vi "Wait Return.vi"(8 "entrée d'erreur (pas d'erreur)":errorcluster, 10 "Report ?":bool, 11 "Send_Frame en entrée":refnum<class "Nodon_Send_Command_UART.lvclass">) -> (0 "sortie d'erreur":errorcluster, 1 "Send again":bool, 2 "Data":string, 3 "Send_Frame en sortie":refnum<class "Nodon_Send_Command_UART.lvclass">, 4 "Command ID":string, 5 "Command Type":string)   [LabVIEW 2020, in "Library Test.lvlib" / "Nodon_Send_Command_UART.lvclass"]
uses:
  Nodon_Send_Command_UART.lvclass
  C:/Users/ngarcin/OneDrive - Altyor/Standard TB/Class/Test/Test (Default)/Test (Default).lvclass
  Commun VI/TypeDef/Commande UART/Parametre UART.ctl
  UART/UART (Default)/Class UART (Default).lvclass
  JSON API/JSON Value/Set from JSON string.vi
  JSON API/Variant JSON/Variant to JSON.vi
  JSON API/JSON Value/Get Item by name array.vi
  Instrument/Instrument (Default)/Class Instrument (Default).lvclass
  JSON API/JSON Value/JSON Value.lvclass
  Nodon_Send_Command_UART.lvclass/Nodon_Send_Command_UART.ctl
  JSON API/Variant JSON/Variant JSON.lvlib
  JSON API/Get Polymorphic/JSON GetSet.lvlib
  Commun VI/Library Commun.lvlib
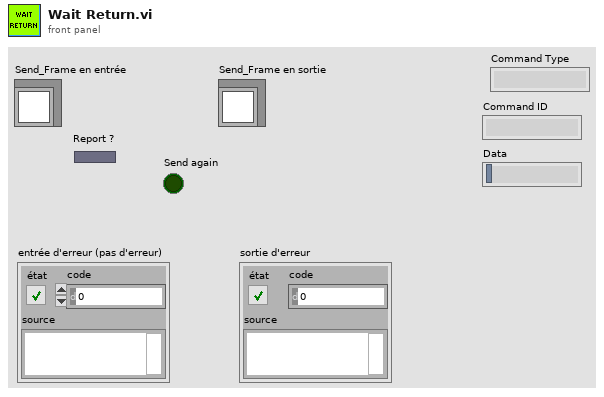
[diagram p1: front panel]
types:
  T1 = typedef "Parametre UART.ctl" = cluster{"Address Device":refnum<visa-resource-name>, "Baud Rate":u32, "Data Bit":u16, "stop bits (10: 1 bit)":u16, "parity (0:none)":enum16{"None", "Odd", "Even", "Mark", "Space"}, "flow control (0:none)":u16, "termination char ":u8, "Enable Termination":bool, "Nb Octet to Read":u16, "Class UART":refnum<class "Class UART (Default).lvclass">}
  T2 = cluster{"Frame Read":string, "Frame received":bool, "Frame NOk":bool}
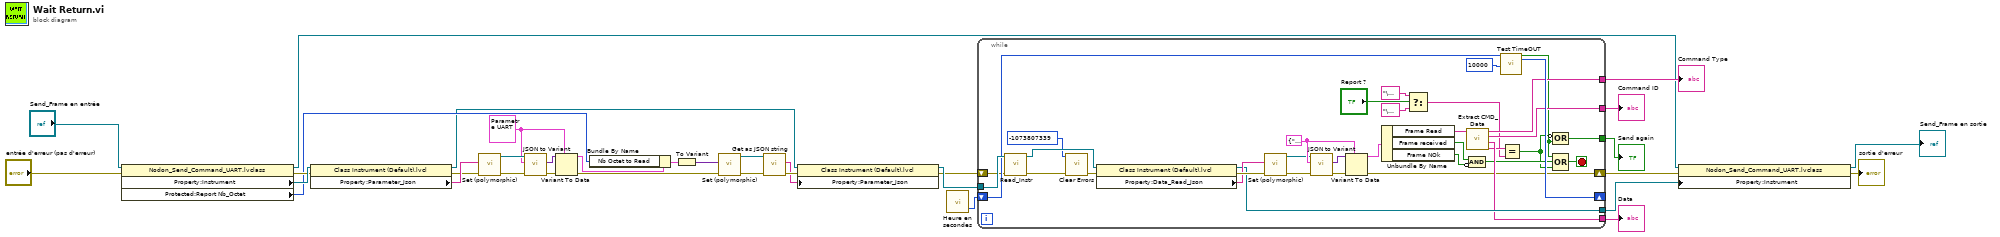
[diagram p0: block diagram]
diagram:
  w14 = T1 {"Address Device"="", "Baud Rate"=0, "Data Bit"=0, "stop bits (10: 1 bit)"=0, "parity (0:none)"=enum."None", "flow control (0:none)"=0, "termination char "=0, "Enable Termination"=FALSE, "Nb Octet to Read"=0, "Class UART"=refnum} ("Parameter")
  n1 = property class="Nodon_Send_Command_UART.lvclass"(reference="Send_Frame en entrée", error in="entrée d'erreur (pas d'erreur)") -> (reference out=w23:refnum<class "Nodon_Send_Command_UART.lvclass">, error out=w15:errorcluster, "Property:Instrument"=w16:refnum<class "Class Instrument (Default).lvclass">, "Protected:Report Nb_Octet"=w12:u16)
  n2 = property class="Class Instrument (Default).lvcl"(reference=w16, error in=w15) -> (reference out=w6:refnum<class "Class Instrument (Default).lvclass">, error out=w17:errorcluster, "Property:Parameter_Json"=w18:string)
  n3 = call-poly "Set (polymorphic).vi"("error in (no error)"=w17, "JSON stream"=w18) -> ("error out"=w20:errorcluster, "JSON Value out"=w22:refnum<class "JSON Value.lvclass">)  [unwired: 7 in, 1 out]
  n4 = call "JSON to Variant.vi"("error in (no error)"=w20, "Variant (Data Type)"=w14, "JSON Value"=w22) -> ("error out"=w21:errorcluster, "Variant out"=w19:variant)  [unwired: 7 in]
  n5 = Variant To Data(error in=w21, type=w14, Variant=w19) -> (data=w13:T1, error out=w8:errorcluster)
  n6 = Bundle By Name(cluster=w13, "Nb Octet to Read"=w12) -> (w7:T1)
  n7 = To Variant(anything=w7) -> (Variant=w11:variant)
  n8 = call-poly "Set (polymorphic).vi"("error in (no error)"=w8, "Variant"=w11) -> ("error out"=w9:errorcluster, "JSON Value out"=w10:refnum<class "JSON Value.lvclass">)  [unwired: 8 in]
  n9 = call "Get as JSON string.vi"("error in (no error)"=w9, "JSON Value in"=w10) -> ("error out"=w4:errorcluster, "<JSON>"=w2:string)  [unwired: 8 in]
  n10 = property class="Class Instrument (Default).lvcl"(reference=w6, error in=w4, "Property:Parameter_Json"=w2) -> (reference out=w5:refnum<class "Class Instrument (Default).lvclass">, error out=w3:errorcluster)
  n11 = call "Heure en secondes.vi"() -> ("Heure en milisecondes"=w1:u32)  [unwired: 2 in, 1 out]
  n12 = while {
    tunnel: w5 -> [w59]
    shift-right: [w50] -> w27
    shift-left: w3 -> [w37]
    tunnel: [w57] -> w24
    shift-right: [w55] -> _
    shift-left: w1 -> [w56]
    tunnel: [w51] -> w33
    tunnel: [w52] -> w32
    tunnel: [w49] -> w31
    tunnel: [w48] -> w30
    stop <- w45 stop-if-true
    w67 = T2 {"Frame Read"="", "Frame received"=FALSE, "Frame NOk"=FALSE}
    n13 = call-dynamic "Read_Instr.vi"("error in (no error)"=w37, "Class Instrument (Default) en entrée"=w59) -> ("error out"=w36:errorcluster, "Class Instrument (Default) en sortie"=w60:refnum<class "Class Instrument (Default).lvclass">)  [unwired: 8 in]
    n14 = call <vilib>:"Clear Errors.vi"("error in (no error)"=w36, "specific error code to clear (0: all)"=-1073807339) -> ("error out"=w34:errorcluster)  [unwired: 4 in, 1 out]
    n15 = property class="Class Instrument (Default).lvcl"(reference=w60, error in=w34) -> (reference out=w57:refnum<class "Class Instrument (Default).lvclass">, error out=w65:errorcluster, "Property:Data_Read_Json"=w64:string)
    n16 = call-poly "Set (polymorphic).vi"("error in (no error)"=w65, "JSON stream"=w64) -> ("error out"=w61:errorcluster, "JSON Value out"=w63:refnum<class "JSON Value.lvclass">)  [unwired: 7 in, 1 out]
    n17 = call "JSON to Variant.vi"("error in (no error)"=w61, "Variant (Data Type)"=w67, "JSON Value"=w63) -> ("error out"=w62:errorcluster, "Variant out"=w66:variant)  [unwired: 7 in]
    n18 = Variant To Data(error in=w62, type=w67, Variant=w66) -> (data=w68:T2, error out=w50:errorcluster)
    n19 = Unbundle By Name(w68) -> ("Frame Read"=w38:string, "Frame received"=w58:bool, "Frame NOk"=w54:bool)
    n20 = Select(t="\u0000" ("cas vrai"), s="Report ?", f="\u0001" ("x")) -> (s? t:f=w41:string)
    n21 = call "Extract CMD_Data.vi"("Frame"=w38) -> ("Frame Type"=w44:string, "DATA"=w51:string, "Command ID"=w49:string, "Command Type"=w48:string)  [unwired: 7 in]
    n22 = Compound Arithmetic op=AND ("Opérateur arithmétique")(w58, invert w54) -> (w47:bool)
    n23 = call "Test TimeOUT.vi"("OLD Time"=w56, "TimeOut ms"=u32 10000) -> ("Timeout ?"=w46:bool, "NEW Time"=w55:u32)  [unwired: 13 in, 3 out]
    n24 = Equal?(x=w44, y=w41) -> (x = y?=w39:bool)
    n25 = Compound Arithmetic op=OR ("Opérateur arithmétique")(invert w39, w46) -> (w52:bool)
    n26 = Compound Arithmetic op=OR ("Opérateur arithmétique")(w46, w47, w39) -> (w45:bool)
  }
  "Data" <- w33
  "Send again" <- w32
  "Command ID" <- w31
  "Command Type" <- w30
  n27 = property class="Nodon_Send_Command_UART.lvclass"(reference=w23, error in=w27, "Property:Instrument"=w24) -> (reference out=→"Send_Frame en sortie":refnum<class "Nodon_Send_Command_UART.lvclass">, error out=→"sortie d'erreur":errorcluster)
